vi "GetParam.vi"(8 "error in (no error)":errorcluster caption="entrée d'erreur (pas d'erreur)", 11 "SparseRandomProjection.lvclass":refnum<class "SparseRandomProjection.lvclass">) -> (0 "error out":errorcluster caption="sortie d'erreur", 2 "SparseRandomProjection":T1={"n_components"="auto", "density"="auto", "eps"=0.1, "dense_output"=FALSE, "random_state"=-1} {"random_state" min=-1; "eps" min=0.0}, 3 "SparseRandomProjection.lvclass":refnum<class "SparseRandomProjection.lvclass">)   [LabVIEW 2020, in "SparseRandomProjection.lvclass"]
doc: "Get Parameters"
uses:
  SparseRandomProjection.lvclass
  SparseRandomProjection.lvclass/SparseRandomProjection.ctl
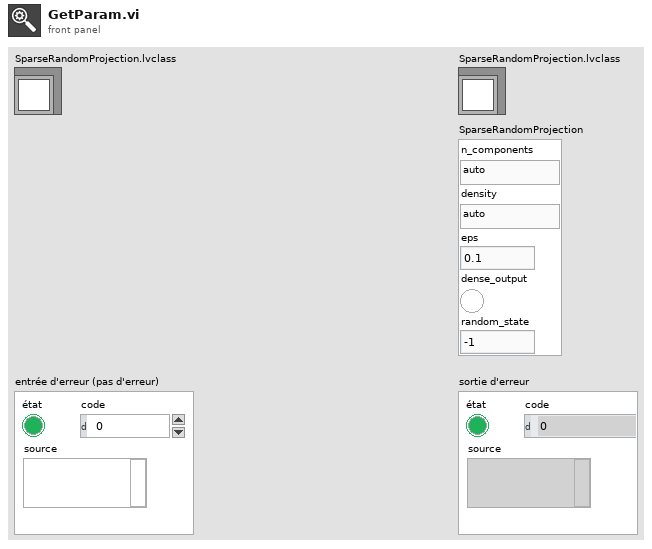
[diagram p1: front panel]
types:
  T1 = cluster{"n_components":string, "density":string, "eps":dbl, "dense_output":bool, "random_state":i32}
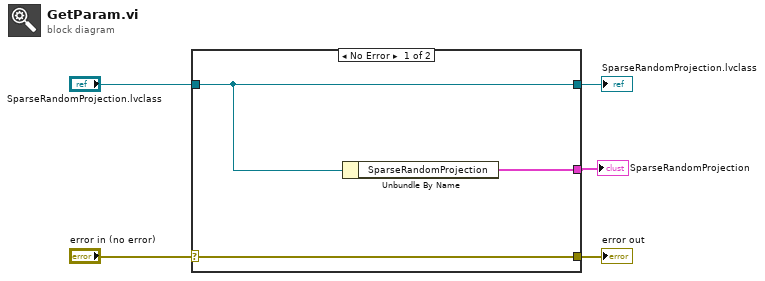
[diagram p0: block diagram]
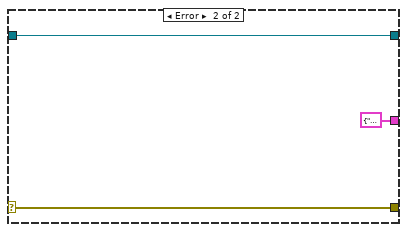
[diagram p2: hidden frame]
diagram:
  n1 = case shown="No Error" "error in (no error)" {
    selector: "error in (no error)" -> [w8 w10]
    tunnel: [w8 w10] -> w4
    tunnel: [w7 w11] -> w2
    tunnel: "SparseRandomProjection.lvclass" -> [w7 w11]
    tunnel: [w6 T1 {"n_components"="", "density"="", "eps"=0.0, "dense_output"=FALSE, "random_state"=0} ("SparseRandomProjection")] -> w1
    frame No Error {
      n2 = Unbundle By Name(w7) -> ("SparseRandomProjection"=w6:T1)
    }
    frame Error {
    }
  }
  "error out" <- w4
  "SparseRandomProjection.lvclass" <- w2
  "SparseRandomProjection" <- w1
